vi "SCCSup Listbox_CheckForSelectedItem.vi"(11 "symbols array":i32[](array[numeric])) -> (1 "checked item index":i32, 3 "item selected?":bool)   [LabVIEW 2017]
doc: "This VI checks the \"checked\" symbol exists in the symbol array. If it does, 0 is returned, Otherwise 2 is returned. The return values are used in the \"Disabled\" control property."
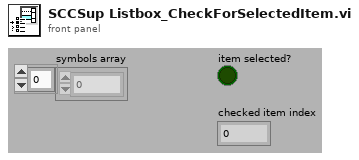
[diagram p1: front panel]
types:
  T1 = enum16{"Get Checked Symbol", "Get Unchecked Symbol", "Toggle Symbol"}
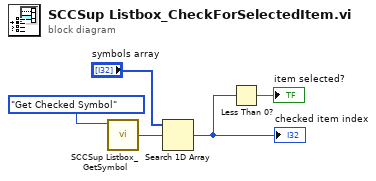
[diagram p0: block diagram]
diagram:
  n1 = call <vilib>:"SCCSup Listbox_GetSymbol.vi"("operation"=T1."Get Checked Symbol") -> ("symbol out"=w4:i32)  [unwired: 6 in]
  n2 = Search 1D Array(1D array="symbols array", element=w4) -> (index of element=w5:i32)  [unwired: 1 in]
  "checked item index" <- w5
  n3 = Less Than 0?(x=w5) -> (x < 0?=→"item selected?":bool)
